vi "Clear_Graphs.vi"(8 "error in (no error)":errorcluster, 11 "Waveform Chart  ref":refnum<vi>) -> (0 "error out":errorcluster, 3 "reference out":refnum<vi>)   [LabVIEW 2024, in "Utilities.lvlib"]
uses:
  Utilities.lvlib
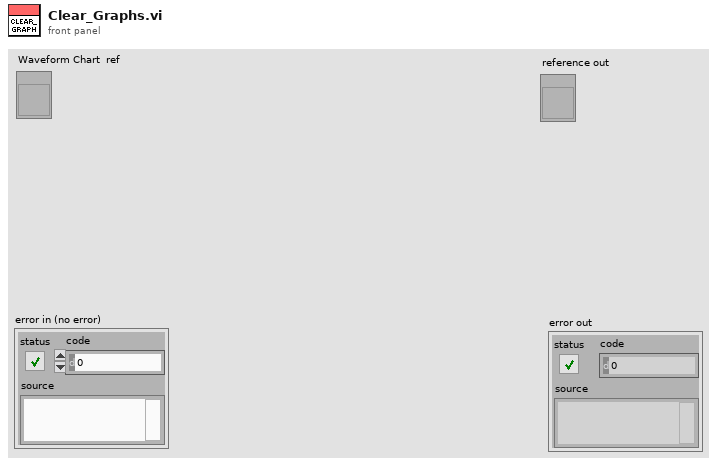
[diagram p1: front panel]
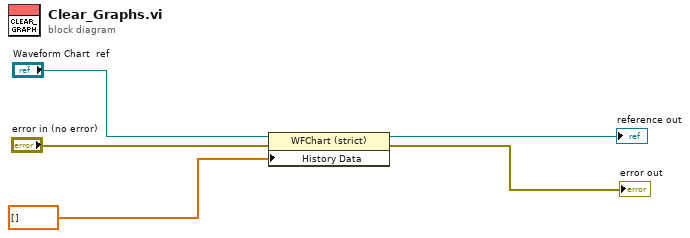
[diagram p0: block diagram]
diagram:
  n1 = property class="WFChart (strict)"(reference="Waveform Chart  ref", error in="error in (no error)", "History Data"=dbl[] []) -> (reference out=→"reference out":refnum<vi>, error out=→"error out":errorcluster)
